vi "Update_ZSpec_Param_Data_SubVI.vi"(11 "output cluster":T1) -> ()   [LabVIEW 2014]
uses:
  <userlib>/Nanonis Prog Interface V5/Nanonis Prog Interface.lvlib
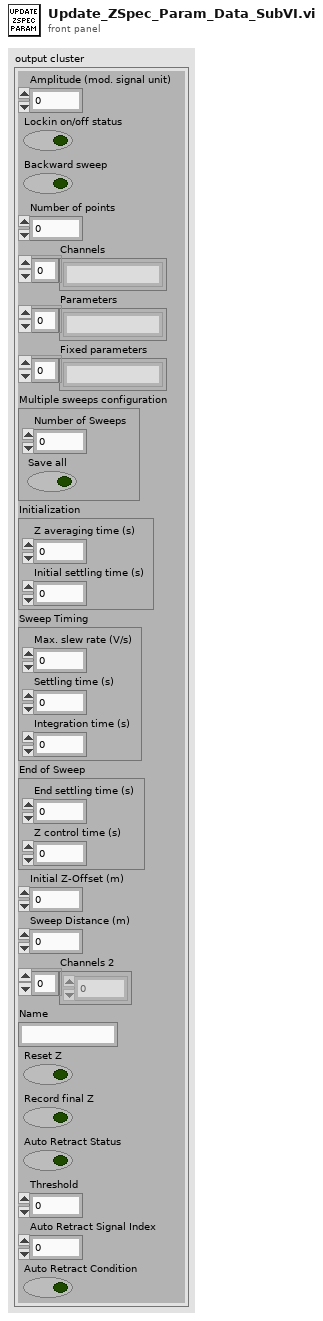
[diagram p1: front panel]
types:
  T1 = cluster{"Amplitude (mod. signal unit)":sgl, "Lockin on/off status":bool, "Backward sweep":bool, "Number of points":i32, "Channels":string[], "Parameters":string[], "Fixed parameters":string[], "Multiple sweeps configuration":cluster{"Number of Sweeps":i32, "Save all":bool}, "Initialization":cluster{"Z averaging time (s)":sgl, "Initial settling time (s)":sgl}, "Sweep Timing":cluster{"Max. slew rate (V/s)":sgl, "Settling time (s)":sgl, "Integration time (s)":sgl}, "End of Sweep":cluster{"End settling time (s)":sgl, "Z control time (s)":sgl}, "Initial Z-Offset (m)":sgl, "Sweep Distance (m)":sgl, "Channels 2":i32[], "Name":string, "Reset Z":bool, "Record final Z":bool, "Auto Retract Status":bool, "Threshold":sgl, "Auto Retract Signal Index":i32, "Auto Retract Condition":bool}
  T2 = cluster{"Z averaging time (s)":sgl, "Initial settling time (s)":sgl}
  T3 = cluster{"Max. slew rate (V/s)":sgl, "Settling time (s)":sgl, "Integration time (s)":sgl}
  T4 = cluster{"End settling time (s)":sgl, "Z control time (s)":sgl}
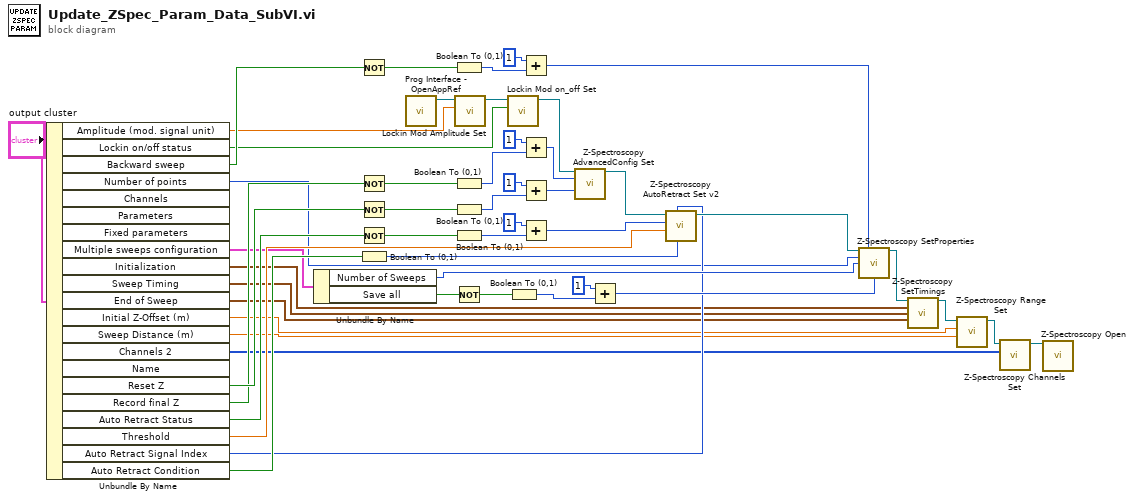
[diagram p0: block diagram]
diagram:
  n1 = Unbundle By Name("output cluster") -> ("Amplitude (mod. signal unit)"=w6:sgl, "Lockin on/off status"=w5:bool, "Backward sweep"=w31:bool, "Number of points"=w18:i32, "Multiple sweeps configuration"=w12:cluster{"Number of Sweeps":i32, "Save all":bool}, "Initialization"=w9:T2, "Sweep Timing"=w8:T3, "End of Sweep"=w7:T4, "Initial Z-Offset (m)"=w15:sgl, "Sweep Distance (m)"=w14:sgl, "Channels 2"=w10:i32[], "Reset Z"=w45:bool, "Record final Z"=w42:bool, "Auto Retract Status"=w23:bool, "Threshold"=w27:sgl, "Auto Retract Signal Index"=w20:i32, "Auto Retract Condition"=w25:bool)  [unwired: 4 out]
  n2 = Unbundle By Name(w12) -> ("Number of Sweeps"=w49:i32, "Save all"=w13:bool)
  n3 = Not(x=w31) -> (.not. x?=w30:bool)
  n4 = Not(x=w42) -> (.not. x?=w39:bool)
  n5 = Not(x=w45) -> (.not. x?=w44:bool)
  n6 = Not(x=w23) -> (.not. x?=w22:bool)
  n7 = Boolean To (0,1)(Boolean=w25) -> (0, 1=w26:i16)
  n8 = call <userlib>:"Prog Interface - OpenAppRef.vi"() -> ("Application reference"=w50:refnum<vi>)  [unwired: 6 in, 1 out]
  n9 = Boolean To (0,1)(Boolean=w30) -> (0, 1=w29:i16)
  n10 = Boolean To (0,1)(Boolean=w39) -> (0, 1=w38:i16)
  n11 = Boolean To (0,1)(Boolean=w44) -> (0, 1=w43:i16)
  n12 = Boolean To (0,1)(Boolean=w22) -> (0, 1=w21:i16)
  n13 = Not(x=w13) -> (.not. x?=w4:bool)
  n14 = call <userlib>:"Lockin Mod Amplitude Set.vi"("Amplitude (mod. signal unit)"=w6, "Application ref in"=w50) -> ("Application ref out"=w1:refnum<vi>)  [unwired: 8 in, 1 out]
  n15 = call <userlib>:"Lockin Mod on_off Set.vi"("Lockin ON/OFF"=w5, "Application ref in"=w1) -> ("Application ref out"=w37:refnum<vi>)  [unwired: 8 in, 1 out]
  n16 = Boolean To (0,1)(Boolean=w4) -> (0, 1=w2:i16)
  n17 = Add(x=i16 1, y=w29) -> (x+y=w33:i16)
  n18 = Add(x=i16 1, y=w38) -> (x+y=w40:i16)
  n19 = Add(x=i16 1, y=w43) -> (x+y=w47:i16)
  n20 = Add(x=i16 1, y=w21) -> (x+y=w24:i16)
  n21 = call <userlib>:"Z-Spectroscopy AdvancedConfig Set.vi"("Application ref in"=w37, "Record final Z position at the end of the sweep"=w40, "Reset Z at the end of the sweep"=w47) -> ("Application ref out"=w36:refnum<vi>)  [unwired: 11 in, 1 out]
  n22 = Add(x=i16 1, y=w2) -> (x+y=w48:i16)
  n23 = call <userlib>:"Z-Spectroscopy AutoRetract Set v2.vi"("Retract condition"=w26, "Auto retract signal index (-2=no change)"=w20, "Threshold"=w27, "Auto retract"=w24, "Application ref in"=w36) -> ("Application ref out"=w35:refnum<vi>)  [unwired: 5 in, 1 out]
  n24 = call <userlib>:"Z-Spectroscopy SetProperties.vi"("Application ref in"=w35, "Backward sweep"=w33, "Num points"=w18, "Num sweeps"=w49, "Save all sweeps (no change)"=w48) -> ("Application ref out"=w34:refnum<vi>)  [unwired: 9 in, 1 out]
  n25 = call <userlib>:"Z-Spectroscopy SetTimings.vi"("Application ref in"=w34, "Initialization (NaN)"=w9, "Sweep Timing (NaN)"=w8, "End of Sweep (NaN)"=w7) -> ("Application ref out"=w16:refnum<vi>)  [unwired: 10 in, 1 out]
  n26 = call <userlib>:"Z-Spectroscopy Range Set.vi"("Z distance (m)"=w14, "Z offset (m) (NaN=no change)"=w15, "Application ref in"=w16) -> ("Application ref out"=w17:refnum<vi>)  [unwired: 6 in, 1 out]
  n27 = call <userlib>:"Z-Spectroscopy Channels Set.vi"("Channels"=w10, "Application ref in"=w17) -> ("Application ref out"=w11:refnum<vi>)  [unwired: 8 in, 1 out]
  n28 = call <userlib>:"Z-Spectroscopy Open.vi"("Application ref in"=w11) -> ()  [unwired: 13 in, 2 out]
